vi "VcoTest.vi"(0 "ClientRefIn":refnum<k24>, 5 "error in (no error)":errorcluster, 11 "hostName":string="localhost", 13 "portNum":i32=50501) -> (10 "VcoCalibration?(T)":bool, 12 "Elapsed(s)":dbl, 14 "ClientRefOut":refnum<k24>, 19 "error out":errorcluster)   [LabVIEW 2018]
uses:
  C:/RageATE-Tetra/Support/TetraLabGUI/FieldTestClient.dll
  Support/TetraLabGUI/FieldTestClient.dll
panel:
  out "NaN/Path/Refnum?":bool
  out "Strat(s)":dbl format="%.6f"
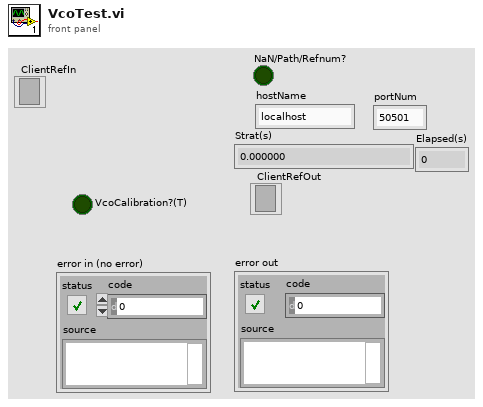
[diagram p1: front panel]
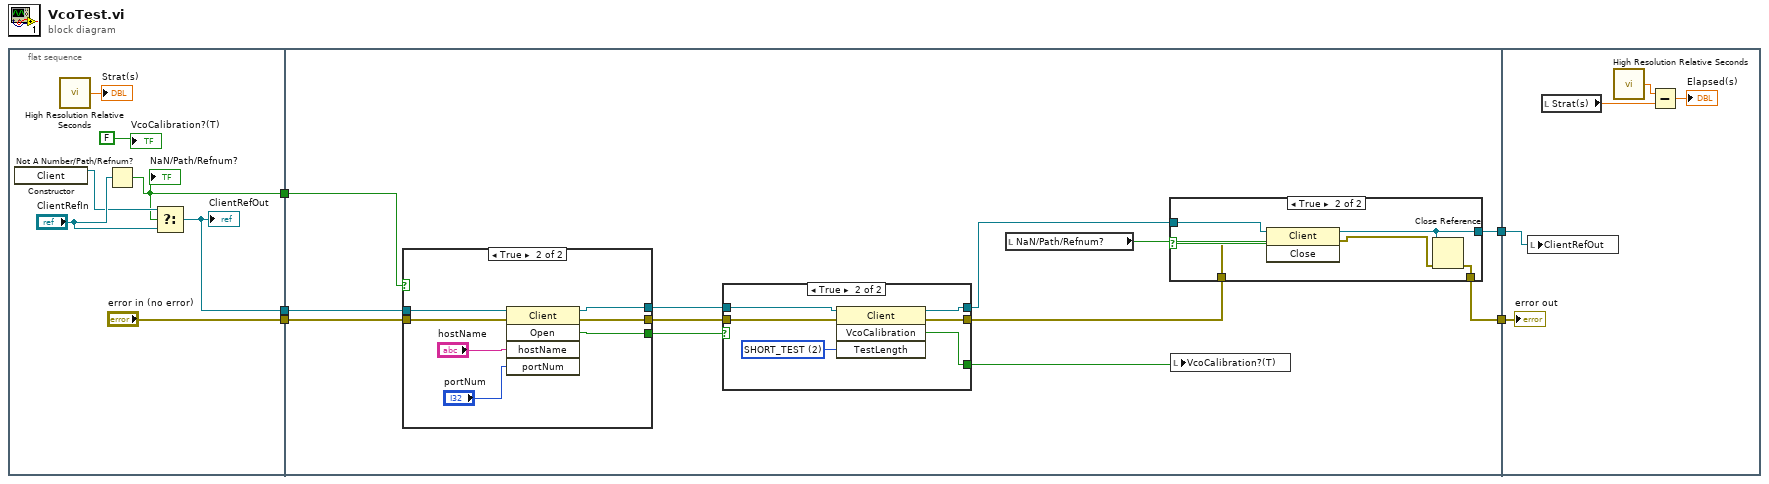
[diagram p0: block diagram]
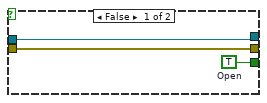
[diagram p2: hidden frame]
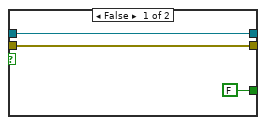
[diagram p4: hidden frame]
diagram:
  n1 = flat-sequence {
    tunnel: ["error in (no error)"] -> w4
    tunnel: [w7] -> w3
    tunnel: [w6] -> w2
    tunnel: [w20] -> w5
    tunnel: w4 -> [w23]
    tunnel: w3 -> [w18]
    tunnel: w2 -> [w17]
    tunnel: [w13] -> w1
    tunnel: w5 -> [w55]
    tunnel: w1 -> [w51]
    frame #0 {
      n2 = constructor class="Client"() -> (reference out=w8:refnum<k24>)  [unwired: 3 in, 2 out]
      n3 = call <vilib>:"High Resolution Relative Seconds.vi"() -> ("relative seconds"=→"Strat(s)":dbl)
      n4 = Not A Number/Path/Refnum?(number/path/refnum="ClientRefIn") -> (NaN/Path/Refnum?=w7:bool)
      "NaN/Path/Refnum?" <- w7
      n5 = Select(t=w8, s=w7, f="ClientRefIn") -> (s? t:f=w6:refnum<k24>)
      "ClientRefOut" <- w6
      "VcoCalibration?(T)" <- FALSE
    }
    frame #1 {
      n6 = case shown="True" w18 {
        tunnel: w23 -> [w27 w34]
        tunnel: [w26 w31] -> w22
        tunnel: [w25 w30] -> w16
        tunnel: [w27 w29] -> w21
        tunnel: w17 -> [w26 w28]
        frame False {
          w25 = TRUE  # Open
        }
        frame True {
          n7 = invoke class="Client" method="Open"(reference=w28, error in=w34, "hostName"="hostName", "portNum"="portNum") -> (reference out=w31:refnum<k24>, error out=w29:errorcluster, "Open"=w30:bool)  [unwired: 1 in, 2 out]
        }
      }
      n8 = case shown="True" w16 {
        tunnel: w22 -> [w43 w49]
        tunnel: [w44 w48] -> w14
        tunnel: w21 -> [w44 w47]
        tunnel: [w43 w46] -> w15
        tunnel: [FALSE ("VcoCalibration") w45] -> w24
        frame False {
        }
        frame True {
          w50 = 2 items=["FULL_TEST"=1, "SHORT_TEST"=2] ("TestLength")
          n9 = invoke class="Client" method="VcoCalibration"(reference=w49, error in=w47, "TestLength"=w50) -> (reference out=w46:refnum<k24>, error out=w48:errorcluster, "VcoCalibration"=w45:bool)  [unwired: 1 in, 1 out]
        }
      }
      n10 = local read "NaN/Path/Refnum?"() -> (w19:bool)
      n11 = case shown="True" w19 {
        tunnel: [w36 w41] -> w20
        tunnel: w15 -> [w35 w40]
        tunnel: w14 -> [w36 w39]
        tunnel: [w35 w37] -> w13
        frame False {
        }
        frame True {
          n12 = invoke class="Client" method="Close"(reference=w40, error in=w39) -> (reference out=w37:refnum<k24>, error out=w38:errorcluster)  [unwired: 1 in, 1 out]
          n13 = Close Reference(reference=w37, error in (no error)=w38) -> (error out=w41:errorcluster)
        }
      }
      n14 = local write "VcoCalibration?(T)"(w24) -> ()
    }
    frame #2 {
      n15 = local write "ClientRefOut"(w51) -> ()
      n16 = local read "Strat(s)"() -> (w53:dbl)
      n17 = call <vilib>:"High Resolution Relative Seconds.vi"() -> ("relative seconds"=w54:dbl)
      n18 = Subtract(x=w54, y=w53) -> (x-y=→"Elapsed(s)":dbl)
      "error out" <- w55
    }
  }
